vi "XML.Sequences.Generate.vi"(8 "error in":errorcluster, 9 "Root name":string="HWConfigFile", 10 "Array":T1[](array[typedef]), 11 "XML file path":path=path "C:/Projects/TM-OS/trunk/Design/XML_HW_config2.xml") -> (0 "error out":errorcluster)   [LabVIEW 2019, in "Tools.lvlib"]
uses:
  Tools.lvlib
  LibXML/LibXML.lvlib
  Modules/Sequences_Management/Gui/Sequences_Management.Gui.Product.ctl
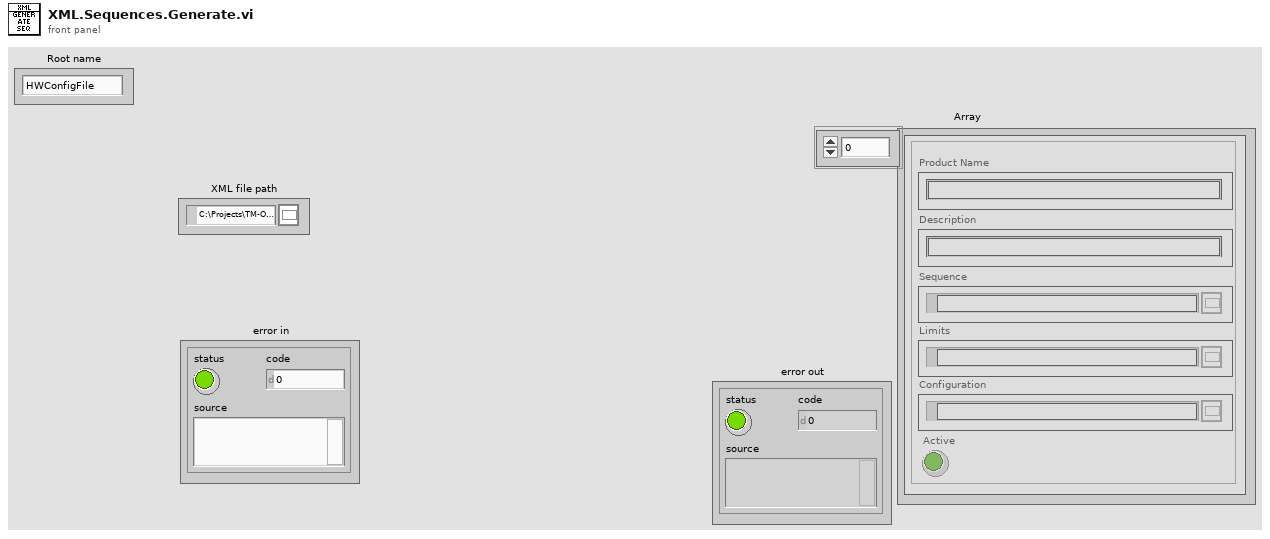
[diagram p1: front panel]
types:
  T1 = typedef "Sequences_Management.Gui.Product.ctl" = cluster{"Product Name":string, "Description":string, "Sequence":path, "Limits":path, "Configuration":path, "Active":bool}
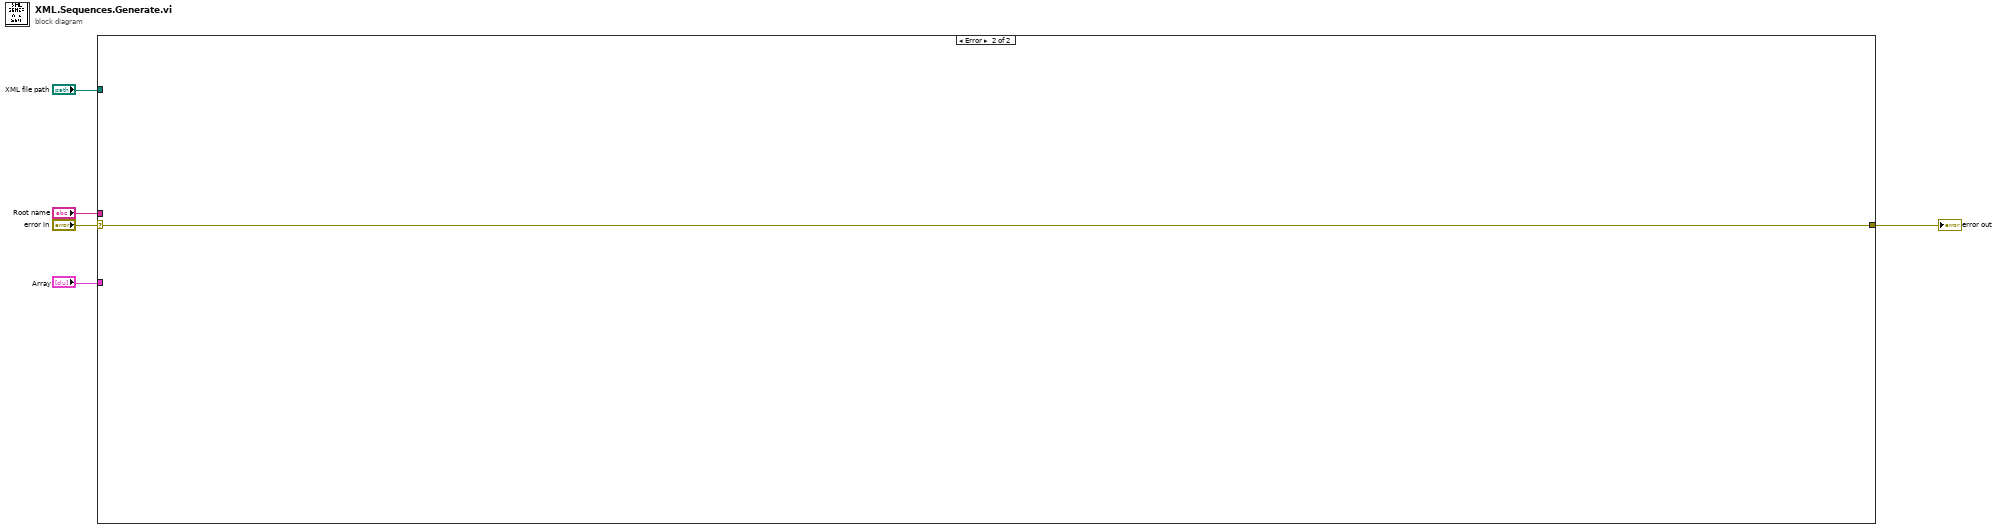
[diagram p0: block diagram]
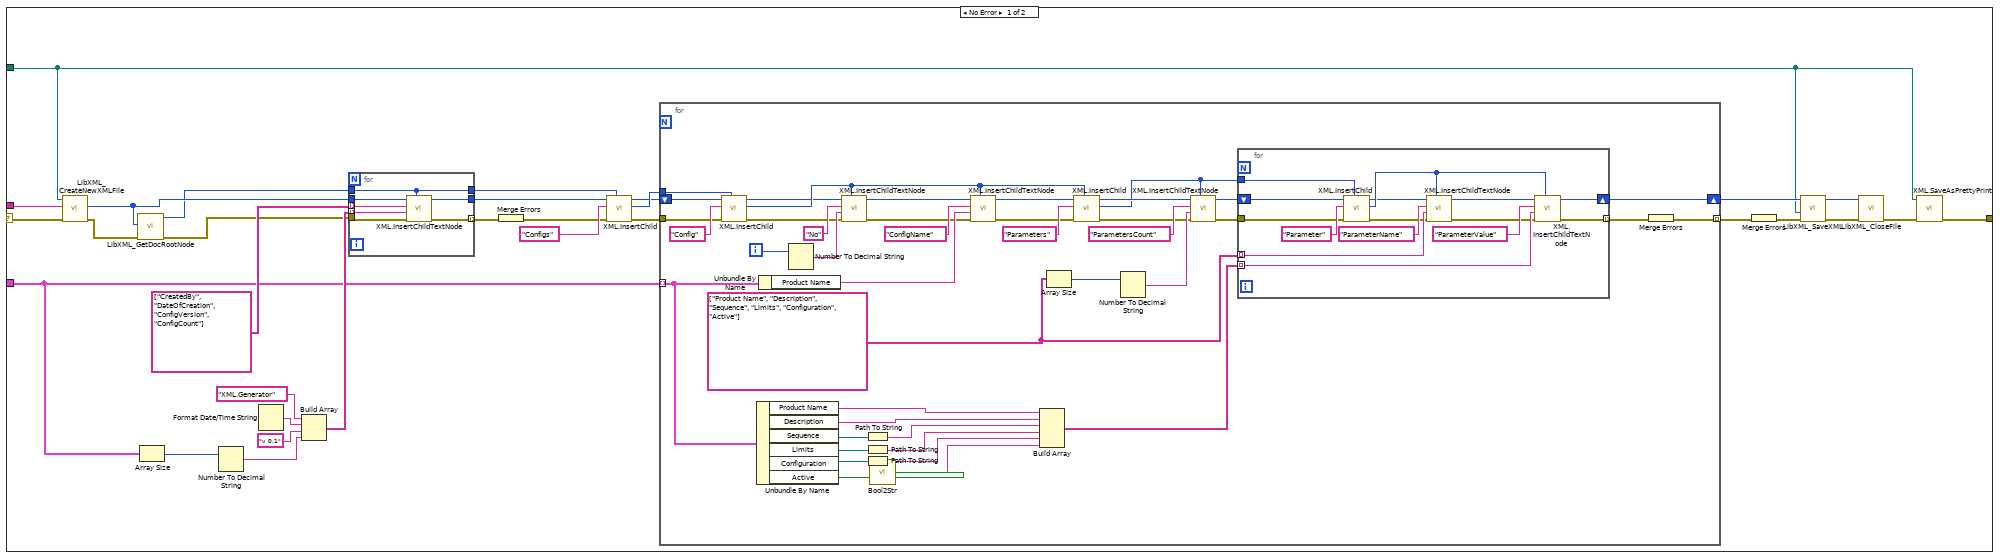
[diagram p2: hidden frame]
diagram:
  n1 = case shown="Error" "error in" {
    selector: "error in" -> [w22 w99]
    tunnel: "Array" -> [w23 _]
    tunnel: "Root name" -> [w21 _]
    tunnel: "XML file path" -> [w7 _]
    tunnel: [w6 w99] -> w1
    frame No Error {
      n2 = call "LibXML_CreateNewXMLFile.vi"("error in"=w22, "Root element name"=w21, "file path"=w7) -> ("error out"=w18:errorcluster, "new doc out"=w20:u32)  [unwired: 6 in, 1 out]
      n3 = call "LibXML_GetDocRootNode.vi"("error in"=w18, "doc"=w20) -> ("error out"=w17:errorcluster, "root node out"=w19:u32)  [unwired: 8 in]
      n4 = Array Size(array=w23) -> (size(s)=w30:i32)
      n5 = Number To Decimal String(number=w30) -> (decimal integer string=w29:string)  [unwired: 1 in]
      n6 = Format Date/Time String() -> (date/time string=w32:string)  [unwired: 3 in]
      n7 = Build Array("XML.Generator" ("Tag Name"), w32, "v 0.1" ("element"), w29) -> (w33:string[])
      n8 = for {
        tunnel: string[] ["CreatedBy", "DateOfCreation", "ConfigVersion", "ConfigCount"] -> [w42] mode=indexing
        tunnel: w20 -> [w39]
        tunnel: w19 -> [w38]
        tunnel: w33 -> [w41] mode=indexing
        tunnel: [w40] -> w26
        tunnel: [w38] -> w24
        tunnel: w17 -> [w37]
        tunnel: [w36] -> w16 mode=indexing
        n9 = call "XML.InsertChildTextNode.vi"("parent"=w38, "error in"=w37, "text"=w41, "name"=w42, "doc"=w39) -> ("error out"=w36:errorcluster, "doc out"=w40:u32)  [unwired: 5 in]
      }
      n10 = Merge Errors(w16) -> (w15:errorcluster)
      n11 = call "XML.InsertChild.vi"("parent"=w24, "error in"=w15, "name"="Configs" ("Tag Name"), "doc"=w26) -> ("error out"=w14:errorcluster, "new node"=w28:u32, "doc out"=w25:u32)  [unwired: 5 in]
      n12 = for {
        tunnel: w23 -> [w63] mode=indexing
        tunnel: w28 -> [w82]
        shift-right: [w80] -> w11
        shift-left: w25 -> [w81]
        tunnel: w14 -> [w50]
        tunnel: [w43] -> w13 mode=indexing
        i -> [w83]
        w54 = string[] ["Product Name", "Description", "Sequence", "Limits", "Configuration", "Active"]
        n13 = call "XML.InsertChild.vi"("parent"=w82, "error in"=w50, "name"="Config" ("Tag Name"), "doc"=w81) -> ("error out"=w49:errorcluster, "new node"=w71:u32, "doc out"=w68:u32)  [unwired: 5 in]
        n14 = Unbundle By Name(w63) -> ("Product Name"=w62:string, "Description"=w61:string, "Sequence"=w60:path, "Limits"=w59:path, "Configuration"=w58:path, "Active"=w52:bool)
        n15 = Unbundle By Name(w63) -> ("Product Name"=w64:string)
        n16 = Number To Decimal String(number=w83) -> (decimal integer string=w78:string)  [unwired: 1 in]
        n17 = call "XML.InsertChildTextNode.vi"("parent"=w71, "error in"=w49, "text"=w78, "name"="No" ("Tag Name"), "doc"=w68) -> ("error out"=w48:errorcluster, "doc out"=w67:u32)  [unwired: 5 in]
        n18 = Path To String(path=w60) -> (string=w57:string)
        n19 = Path To String(path=w59) -> (string=w56:string)
        n20 = Path To String(path=w58) -> (string=w55:string)
        n21 = call "Bool2Str.vi"("Boolean"=w52) -> ("string"=w51:string)
        n22 = call "XML.InsertChildTextNode.vi"("parent"=w71, "error in"=w48, "text"=w64, "name"="ConfigName", "doc"=w67) -> ("error out"=w47:errorcluster, "doc out"=w69:u32)  [unwired: 5 in]
        n23 = Build Array(w62, w61, w57, w56, w55, w51) -> (w53:string[])
        n24 = Array Size(array=w54) -> (size(s)=w75:i32)
        n25 = call "XML.InsertChild.vi"("parent"=w71, "error in"=w47, "name"="Parameters" ("Tag Name"), "doc"=w69) -> ("error out"=w46:errorcluster, "new node"=w65:u32, "doc out"=w70:u32)  [unwired: 5 in]
        n26 = Number To Decimal String(number=w75) -> (decimal integer string=w74:string)  [unwired: 1 in]
        n27 = call "XML.InsertChildTextNode.vi"("parent"=w65, "error in"=w46, "text"=w74, "name"="ParametersCount", "doc"=w70) -> ("error out"=w45:errorcluster, "doc out"=w66:u32)  [unwired: 5 in]
        n28 = for {
          tunnel: w65 -> [w95]
          shift-right: [w90] -> w80
          shift-left: w66 -> [w94]
          tunnel: w54 -> [w89] mode=indexing
          tunnel: w53 -> [w88] mode=indexing
          tunnel: w45 -> [w87]
          tunnel: [w84] -> w44 mode=indexing
          n29 = call "XML.InsertChild.vi"("parent"=w95, "error in"=w87, "name"="Parameter" ("Tag Name"), "doc"=w94) -> ("error out"=w86:errorcluster, "new node"=w93:u32, "doc out"=w92:u32)  [unwired: 5 in]
          n30 = call "XML.InsertChildTextNode.vi"("parent"=w93, "error in"=w86, "text"=w89, "name"="ParameterName", "doc"=w92) -> ("error out"=w85:errorcluster, "doc out"=w91:u32)  [unwired: 5 in]
          n31 = call "XML.InsertChildTextNode.vi"("parent"=w93, "error in"=w85, "text"=w88, "name"="ParameterValue", "doc"=w91) -> ("error out"=w84:errorcluster, "doc out"=w90:u32)  [unwired: 5 in]
        }
        n32 = Merge Errors(w44) -> (w43:errorcluster)
      }
      n33 = Merge Errors(w13) -> (w12:errorcluster)
      n34 = call "LibXML_SaveXML.vi"("error in"=w12, "file path (dialog if empty)"=w7, "doc"=w11) -> ("error out"=w9:errorcluster, "doc copy out"=w10:u32)  [unwired: 6 in, 1 out]
      n35 = call "LibXML_CloseFile.vi"("error in"=w9, "doc"=w10) -> ("error out"=w8:errorcluster)  [unwired: 9 in]
      n36 = call "XML.SaveAsPrettyPrint.vi"("error in (no error)"=w8, "XML file path"=w7) -> ("error out"=w6:errorcluster)  [unwired: 9 in]
    }
    frame Error {
    }
  }
  "error out" <- w1
